vi "Mod_OFDM_ADD_DELETE_Frame.vi"(0 "Configuration in":variant, 2 "OFDM SYmbol Pool":string[](array[string]), 7 "Add/delete":bool, 11 "error in":errorcluster, 12 "Edit Position":cluster{"Row":i32, "Column":i32}, 13 "Config OFDM Frame":T6) -> (4 "Configuration out":variant, 15 "error out":errorcluster)   [LabVIEW 2010]
uses:
  Controls(Type_DEf)/Attribute Data Types.ctl
  Controls(Type_DEf)/Configure Pulse Shaping.ctl
  Controls(Type_DEf)/Pool of Modulator Control.ctl
  Controls(Type_DEf)/Pool of Data Source Control.ctl
  Controls(Type_DEf)/Attribute Names.ctl
  Polymorphic_Sub_VI's/Mod_OFDM_Set_Ofdm_Frame.vi
panel:
  in  "Attribute Data Types":T1={"Pulse Shaping"={"System Filter"={"TX Filter"=enum."none", "Alpha"=0.0, "filter length"=0}, "Modulation system parameters"={"samples per symbol (16)"=0}, "symbol rate (Hz)"=0.0}, "FRAME Table"=[], "OFDM Frame"=[], "Sub Carrier Selection"={"Sub Carrier Selection"=[], "OFDM Parameters"={"# of Sub Carrier"=0, "Length Of Cylic Prefix"=0}}, "Symbol Table"=[], "Symbol Pool"=[], "Pool of Modulators"=[], "Pool of Data Sources"=[], "Atribute Names"={"Data Source Pool"="Data Source Pool ", "Modulator Source Pool"="Modulator Source Pool ", "OFDM SYMBOL POOL"="OFDM SYMBOL POOL", "Symbol Table"="Symbol Table", "Sub Carrier Selection"="Sub Carrier Selection", "OFDM Frame"="OFDM Frame", "FRAME Table"="FRAME Table", "Pulse Shaping"="Pulse Shaping"}} {"Pool of Data Sources"."Register Initial State" format="%08x"; "Pulse Shaping"."symbol rate (Hz)" min=1.0 step=1.0 format="%.2p"; "Pulse Shaping"."Modulation system parameters"."samples per symbol (16)" step=2; "Pulse Shaping"."System Filter"."Alpha" min=0.0 max=1.0 step=0.05 format="%.2f"}
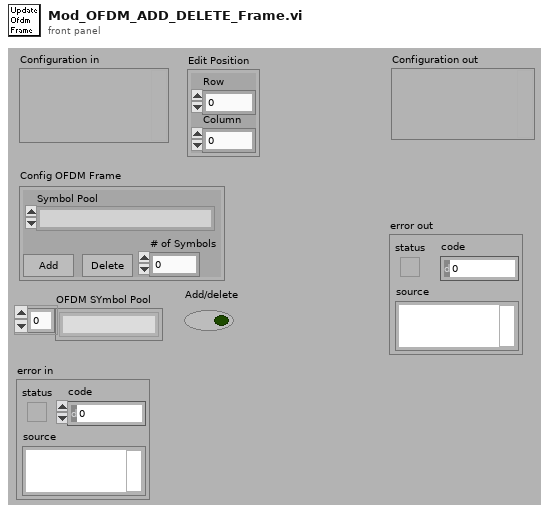
[diagram p1: front panel]
types:
  T1 = typedef "Attribute Data Types.ctl" = cluster{"Pulse Shaping":T2, "FRAME Table":string[][], "OFDM Frame":cluster{"Symbol Name":string, "# of Symbols":i32}[], "Sub Carrier Selection":cluster{"Sub Carrier Selection":cluster{"Sub Carrier":bool, "Data Source":u16, "Modulator":u16}[], "OFDM Parameters":cluster{"# of Sub Carrier":i32, "Length Of Cylic Prefix":i32}}, "Symbol Table":string[][], "Symbol Pool":string[], "Pool of Modulators":T3, "Pool of Data Sources":T4, "Atribute Names":T5}
  T2 = typedef "Configure Pulse Shaping.ctl" = cluster{"System Filter":cluster{"TX Filter":enum16{"none", "Raised Cosine", "Root Raised Cos"}, "Alpha":dbl, "filter length":i32}, "Modulation system parameters":cluster{"samples per symbol (16)":u32}, "symbol rate (Hz)":dbl}
  T3 = typedef "Pool of Modulator Control.ctl" = cluster{"M-QAM":enum16{"4", "16", "64", "256"}, "M-PSK":enum16{"2", "4", "8", "16", "32", "64", "128", "256"}, "Type of Modulation":enum16{"PSK", "QAM"}, " PSK":cluster{"differential PSK":enum16{"disable", "enable"}, "PSK type":enum16{"normal", "shifted", "offset"}}}[]
  T4 = typedef "Pool of Data Source Control.ctl" = cluster{"mode (PN)":enum16{"PN", "pattern", "user"}, "PN sequence order (9)":i32, "Invert Output Bits":enum16{"No", "Yes"}, "Register Initial State ":u32, "User base bit pattern":i8[], "base bit pattern (00001111)":enum16{"0", "1", "01", "0011", "00001111"}, "Reset to Initial State":enum16{"Every OFDM Frame", "Every OFDM Symbol", "Every Sub Carrier"}}[]
  T5 = typedef "Attribute Names.ctl" = cluster{"Data Source Pool":string, "Modulator Source Pool":string, "OFDM SYMBOL POOL":string, "Symbol Table":string, "Sub Carrier Selection":string, "OFDM Frame":string, "FRAME Table":string, "Pulse Shaping":string}
  T6 = cluster{"Symbol Pool":u16, "Add":bool, "Delete":bool, "# of Symbols":u32}
  T7 = cluster{"Symbol Name":string, "# of Symbols":i32}
  T8 = cluster{"Symbol Name":string, "# of Symbols":i32}[]
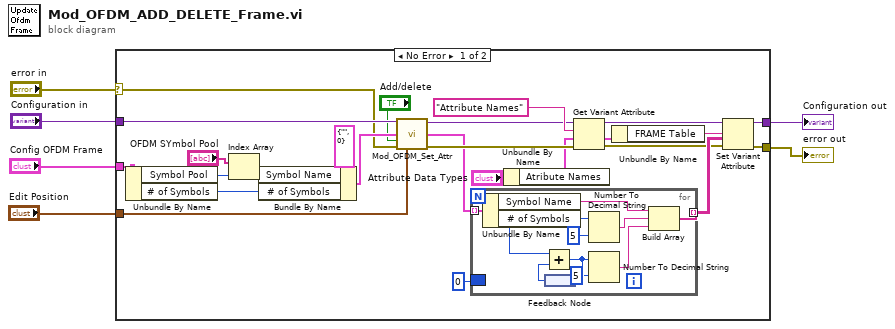
[diagram p0: block diagram]
diagram:
  n1 = case shown="No Error" "error in" {
    selector: "error in" -> [w17 w42]
    tunnel: "Config OFDM Frame" -> [w31 _]
    tunnel: "Configuration in" -> [w18 _]
    tunnel: [w25 w42] -> w4
    tunnel: [w23 _] -> w3
    tunnel: "Edit Position" -> [w8 _]
    frame No Error {
      n2 = Unbundle By Name(w31) -> ("Symbol Pool"=w30:u16, "# of Symbols"=w27:u32)
      n3 = Index Array(array="OFDM SYmbol Pool", index=w30) -> (element=w26:string)
      n4 = Bundle By Name(cluster=T7 {"Symbol Name"="", "# of Symbols"=0}, "Symbol Name"=w26, "# of Symbols"=w27) -> (w19:T7)
      n5 = call-poly "Mod_OFDM_Set_Attr.vi"("Configure Variant"=w18, "ADD Symbol"=w19, "Add/delete"="Add/delete", "error in"=w17, "Edit Position"=w8) -> ("Configure Variant"=w15:variant, "OFDM Frame"=w12:T8, "error out"=w16:errorcluster)  [unwired: 8 in]
      n6 = for {
        tunnel: w12 -> [w41] mode=indexing
        tunnel: [w38] -> w24 mode=indexing
        border: 0 -> [_]
        n7 = Unbundle By Name(w41) -> ("Symbol Name"=w40:string, "# of Symbols"=w37:i32)
        n8 = feedback #1() -> (w36:i32)
        n9 = Add(x=w37, y=w36) -> (x+y=w35:i32)
        n10 = feedback-in #1(w35) -> ()
        n11 = Number To Decimal String(number=w37, width (-)=i16 5) -> (decimal integer string=w39:string)
        n12 = Number To Decimal String(number=w35, width (-)=i16 5) -> (decimal integer string=w34:string)
        n13 = Build Array(w40, w39, w34) -> (w38:string[])
      }
      n14 = Unbundle By Name("Attribute Data Types") -> ("Atribute Names"=w13:T5)
      n15 = Get Variant Attribute(Variant=w15, name="Attribute Names", default value (empty Variant)=w13, error in=w16) -> (duplicate Variant=w11:variant, value=w21:T5, error out=w10:errorcluster)  [unwired: 1 out]
      n16 = Unbundle By Name(w21) -> ("FRAME Table"=w20:string)
      n17 = Set Variant Attribute(Variant=w11, name=w20, value=w24, error in=w10) -> (Variant out=w23:variant, error out=w25:errorcluster)  [unwired: 1 out]
    }
    frame Error {
    }
  }
  "Configuration out" <- w3
  "error out" <- w4
